vi "Home.vi"() -> ()   [LabVIEW 2018]
panel:
  in  "Move to home":bool
  in  "MG17Motor B":refnum<k7>(container)
  in  "MG17Motor A":refnum<k7>(container)
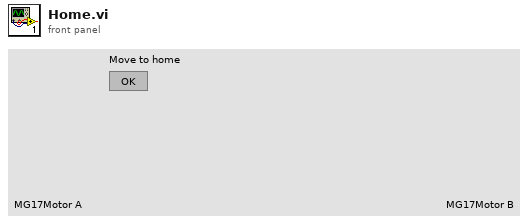
[diagram p1: front panel]
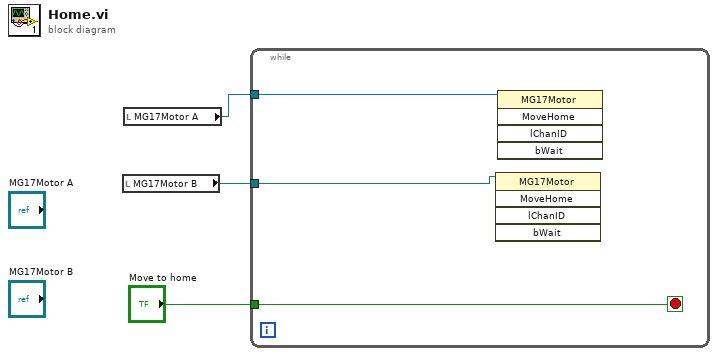
[diagram p0: block diagram]
diagram:
  n1 = local read "MG17Motor B"() -> (w3:refnum<k7>)
  n2 = local read "MG17Motor A"() -> (w2:refnum<k7>)
  n3 = while {
    tunnel: w3 -> [w5]
    tunnel: w2 -> [w6]
    tunnel: "Move to home" -> [w4]
    stop <- w4 stop-if-true
    n4 = invoke class="MG17Motor" method="MoveHome"(reference=w5) -> ()  [unwired: 3 in, 6 out]
    n5 = invoke class="MG17Motor" method="MoveHome"(reference=w6) -> ()  [unwired: 3 in, 6 out]
  }
